vi "Endpoints.vi"(10 "Array":dbl[](array[numeric])) -> (2 "One-Half Engpoints Sum":dbl format="%.6g")   [LabVIEW 2017]
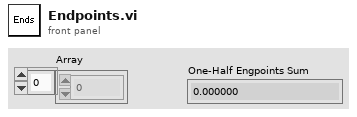
[diagram p1: front panel]
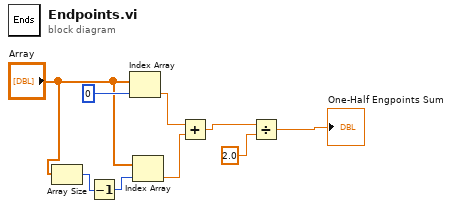
[diagram p0: block diagram]
diagram:
  n1 = Array Size(array="Array") -> (size(s)=w8:i32)
  n2 = Decrement(x=w8) -> (x-1=w6:i32)
  n3 = Index Array(array="Array", index=0) -> (element=w5:dbl)
  n4 = Index Array(array="Array", index=w6) -> (element=w4:dbl)
  n5 = Add(x=w5, y=w4) -> (x+y=w2:dbl)
  n6 = Divide(x=w2, y=2.0) -> (x/y=→"One-Half Engpoints Sum":dbl)
